vi "Steer_Utilitiy.vi"(9 "Right":bool, 10 "Left":bool, 11 "array":bool[](array[boolean])) -> (1 "Right":bool, 2 "Left":bool, 3 "Steer Position":dbl)   [LabVIEW 2015]
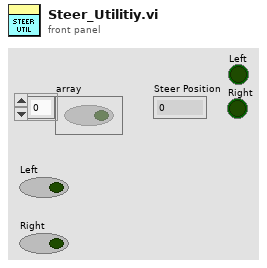
[diagram p1: front panel]
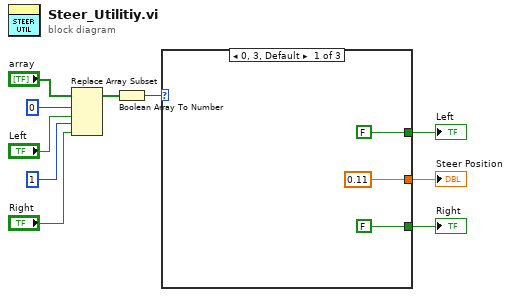
[diagram p0: block diagram]
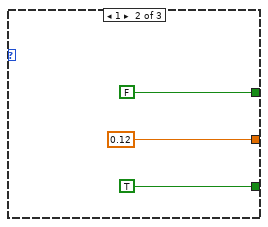
[diagram p2: hidden frame]
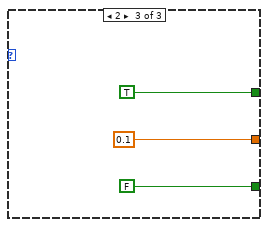
[diagram p3: hidden frame]
diagram:
  n1 = Replace Array Subset(array="array", new element #1="Left", index #1=0 ("index"), new element #2="Right", index #2=1 ("index")) -> (w7:bool[])
  n2 = Boolean Array To Number(Boolean array=w7) -> (number=w8:u32)
  n3 = case shown="0, 3, Default" w8 {
    tunnel: [0.11 0.12 0.1] -> w9
    tunnel: [FALSE FALSE TRUE] -> w2
    tunnel: [FALSE TRUE FALSE] -> w1
    frame 0, 3, Default {
    }
    frame 1 {
    }
    frame 2 {
    }
  }
  "Steer Position" <- w9
  "Left" <- w2
  "Right" <- w1
